vi "Acquire_OSCILL_SubVI_vSingle.vi"(4 "mV/div [CH2]":dbl=5.0, 8 "error in (no error)":errorcluster, 11 "VISA resource name":refnum<visa-resource-name>) -> (0 "error out":errorcluster, 1 "Time":dbl[](array[numeric]), 3 "CH1_averaged":dbl[](array[numeric]), 5 "VISA resource name out":refnum<visa-resource-name>)   [LabVIEW 2017]
uses:
  Agilent 2000 3000 X-Series/Agilent 2000 3000 X-Series.lvlib
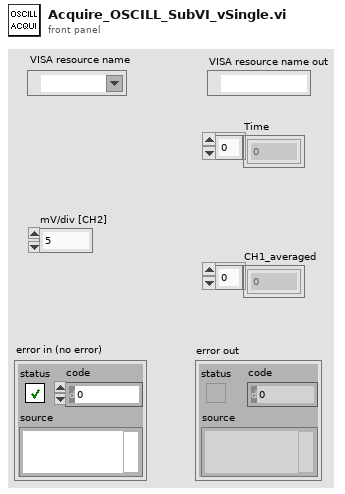
[diagram p1: front panel]
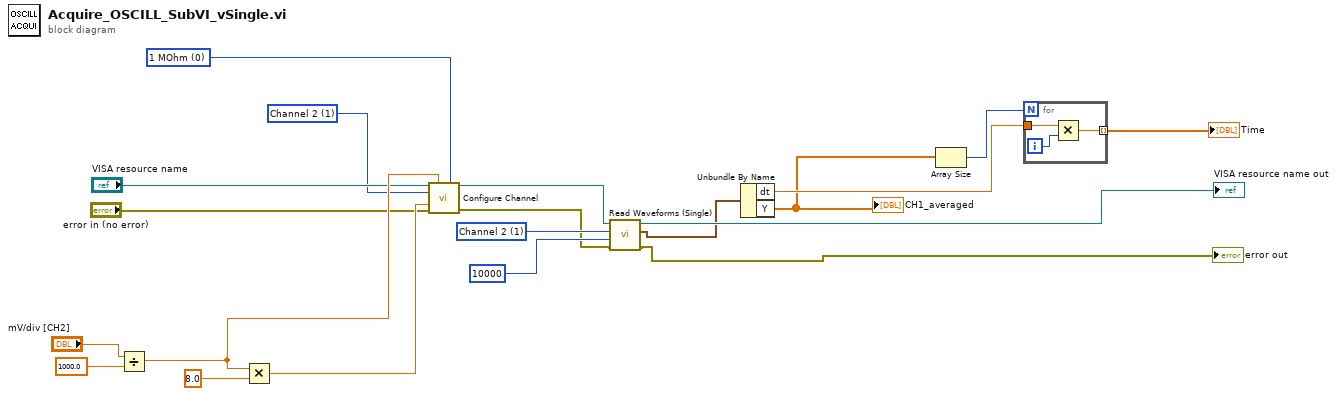
[diagram p0: block diagram]
diagram:
  w3 = 1 items=["Channel 1", "Channel 2", "Channel 3", "Channel 4"] ("Channel Name (0: Channel 1)")
  w15 = 0 items=["1 MOhm", "50 Ohm"] ("Impedance (0: 1 MOhm)")
  w6 = 1 items=["Channel 1"=0, "Channel 2"=1, "Channel 3"=2, "Channel 4"=3, "Digital Bus Low"=9, "Digital Bus High"=10] ("Source Channel (0: Channel 1)")
  n1 = Divide(x="mV/div [CH2]", y=1000.0) -> (x/y=w16:dbl)
  n2 = Multiply(x=w16, y=8.0) -> (x*y=w17:dbl)
  n3 = call "Configure Channel.vi"("VISA resource name"="VISA resource name", "Vertical Scale (5.0 V)"=w16, "Impedance (0: 1 MOhm)"=w15, "Channel Name (0: Channel 1)"=w3, "Vertical Range (40.0 V)"=w17, "error in (no error)"="error in (no error)") -> ("VISA resource name out"=w2:refnum<visa-resource-name>, "error out"=w1:errorcluster)  [unwired: 5 in, 3 out]
  n4 = call "Read Waveforms (Single).vi"("error in (no error)"=w1, "Timeout (10000 ms)"=u32 10000 ("y"), "Source Channel (0: Channel 1)"=w6, "VISA resource name"=w2) -> ("error out"=→"error out":errorcluster, "Waveform Data"=w7:waveform(dbl), "VISA resource name out"=→"VISA resource name out":refnum<visa-resource-name>)  [unwired: 1 in, 4 out]
  n5 = Unbundle By Name(w7) -> ("dt"=w13:dbl, "Y"=w11:dbl[])
  "CH1_averaged" <- w11
  n6 = Array Size(array=w11) -> (size(s)=w14:i32)
  n7 = for {
    N: w14 -> [_]
    tunnel: [w23] -> w12 mode=indexing
    tunnel: w13 -> [w21]
    i -> [w22]
    n8 = Multiply(x=w21, y=w22) -> (x*y=w23:dbl)
  }
  "Time" <- w12
